vi "Get Rel Path Start.vi"(8 "error in (no error)":errorcluster) -> (0 "error out":errorcluster, 3 "appended path":path)   [LabVIEW 2020]
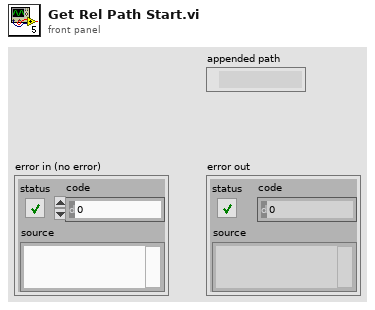
[diagram p1: front panel]
types:
  T1 = enum32{"invalid app kind", "Development System", "Run Time System", "Student Edition", "Embedded LabVIEW", "Evaluation", "Custom"}
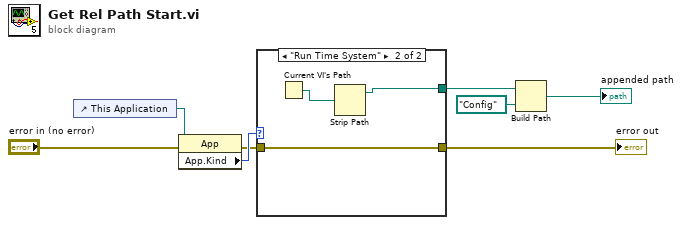
[diagram p0: block diagram]
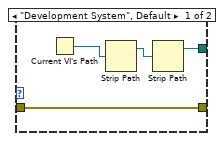
[diagram p2: hidden frame]
diagram:
  n1 = control-ref of="This Application"() -> (w1:refnum<vi>)
  n2 = property class="App"(reference=w1, error in="error in (no error)") -> (error out=w2:errorcluster, "App.Kind"=w3:T1)  [unwired: 1 out]
  n3 = case shown="\"Run Time System\"" w3 {
    tunnel: w2 -> [w9 w13]
    tunnel: [w10 w14] -> w4
    tunnel: [w9 w13] -> w8
    frame "Development System", Default {
      n4 = Current VI's Path() -> (path=w12:path)
      n5 = Strip Path(path=w12) -> (stripped path=w11:path)  [unwired: 1 out]
      n6 = Strip Path(path=w11) -> (stripped path=w10:path)  [unwired: 1 out]
    }
    frame "Run Time System" {
      n7 = Current VI's Path() -> (path=w15:path)
      n8 = Strip Path(path=w15) -> (stripped path=w14:path)  [unwired: 1 out]
    }
  }
  "error out" <- w8
  n9 = Build Path(base path=w4, name or relative path=path "Config") -> (appended path=→"appended path":path)
